vi "3090仪器参数上传.vi"(11 "错误输入（无错误）":errorcluster) -> (15 "error out":errorcluster)   [LabVIEW 2016, in "数据传输系统.lvlib"]
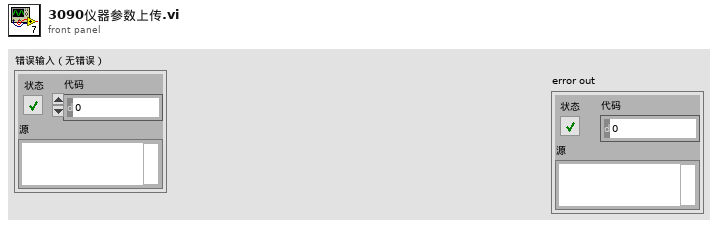
[diagram p1: front panel]
types:
  T1 = cluster{"氨氮仪器参数索引起始时间":string, "总磷仪器参数索引起始时间":string, "总氮仪器参数索引起始时间":string, "CODMn仪器参数索引起始时间":string, "CODCr仪器参数索引起始时间":string, "DO仪器参数索引起始时间":string, "PH仪器参数索引起始时间":string, "比电导率仪器参数索引起始时间":string, "水温仪器参数索引起始时间":string, "浊度仪器参数索引起始时间":string, "叶绿素a仪器参数索引起始时间":string, "藻密度仪器参数索引起始时间":string, "ORP仪器参数索引起始时间":string, "氟化物仪器参数索引起始时间":string, "挥发酚仪器参数索引起始时间":string}
  T2 = cluster{"[0]":string, "[1]":string, "[2]":string, "[3]":string, "[4]":string, "[5]":string, "[6]":string, "[7]":string, "[8]":string, "[9]":string, "[10]":string, "[11]":string, "[12]":string, "[13]":string, "[14]":string}
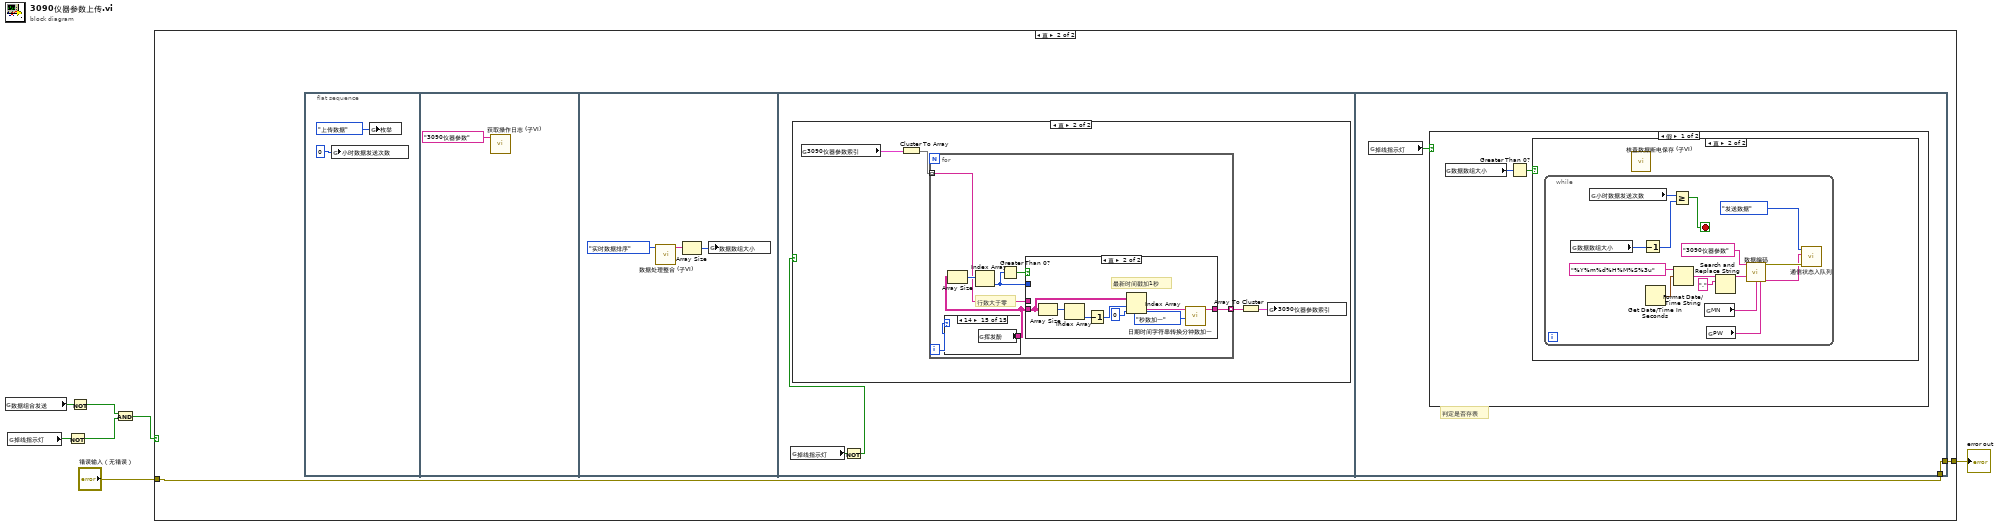
[diagram p0: block diagram]
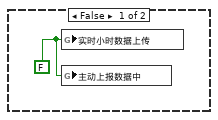
[diagram p2: hidden frame]
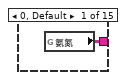
[diagram p4: hidden frame]
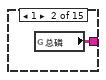
[diagram p5: hidden frame]
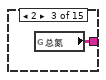
[diagram p6: hidden frame]
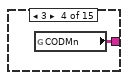
[diagram p7: hidden frame]
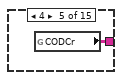
[diagram p8: hidden frame]
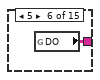
[diagram p9: hidden frame]
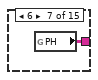
[diagram p10: hidden frame]
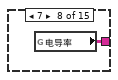
[diagram p11: hidden frame]
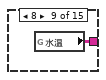
[diagram p12: hidden frame]
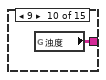
[diagram p13: hidden frame]
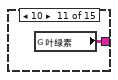
[diagram p14: hidden frame]
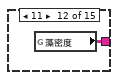
[diagram p15: hidden frame]
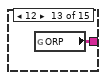
[diagram p16: hidden frame]
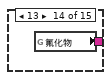
[diagram p17: hidden frame]
diagram:
  n1 = global read "断电保存全局.vi" "数据组合发送"() -> (w4:bool)
  n2 = global read "全局 数据发送重叠.vi" "掉线指示灯"() -> (w7:bool)
  n3 = Not(x=w7) -> (.not. x?=w2:bool)
  n4 = Not(x=w4) -> (.not. x?=w3:bool)
  n5 = And(x=w3, y=w2) -> (x .and. y?=w1:bool)
  n6 = case shown="真" w1 {
    tunnel: [_ w10] -> w6
    tunnel: "错误输入（无错误）" -> [_ w9]
    frame False {
      w8 = FALSE ("小时数据上传")
      n7 = global write "全局1.vi" "实时小时数据上传"(w8) -> ()
      n8 = global write "全局 数据发送重叠.vi" "主动上报数据中"(w8) -> ()
    }
    frame True {
      n9 = flat-sequence {
        tunnel: [w54] -> w10
        tunnel: w9 -> [w54]
        frame #0 {
          n10 = global write "全局 小时数据发送次数.vi" "小时数据发送次数"(0 ("小时数据发送次数")) -> ()
          n11 = global write "全局1.vi" "枚举"(enum16{"返回请求应答", "上传数据", "返回执行结果"}."上传数据" ("枚举")) -> ()
        }
        frame #1 {
          n12 = call "获取操作日志 (子VI).vi"("table输入"="3090仪器参数") -> ()  [unwired: 11 in]
        }
        frame #2 {
          n13 = call "数据处理整合 (子VI).vi"("枚举"=enum16{"实时数据排序", "小时数据排序"}."实时数据排序") -> ("已排序的数组"=w16:string[])  [unwired: 10 in]
          n14 = Array Size(array=w16) -> (size(s)=w15:i32)
          n15 = global write "全局 数据数组大小.vi" "数据数组大小"(w15) -> ()
        }
        frame #3 {
          n16 = global read "全局 数据发送重叠.vi" "掉线指示灯"() -> (w18:bool)
          n17 = Not(x=w18) -> (.not. x?=w17:bool)
          n18 = case shown="真" w17 {
            frame False {
            }
            frame True {
              n19 = global read "全局 时间2.vi" "3090仪器参数索引"() -> (w22:T1)
              n20 = Cluster To Array(cluster=w22) -> (array=w21:string[])
              n21 = for {
                tunnel: [w26] -> w19 mode=indexing
                tunnel: w21 -> [w25] mode=indexing
                i -> [w24]
                # "行数大于零"
                n22 = case shown="14" w24 {
                  tunnel: [w30 w31 w32 w33 w34 w35 w36 w37 w38 w39 w40 w41 w42 w43 w44] -> w23
                  frame 0, Default {
                    n23 = global read "全局 所有参数.vi" "氨氮"() -> (w30:string[][])
                  }
                  frame 1 {
                    n24 = global read "全局 所有参数.vi" "总磷"() -> (w31:string[][])
                  }
                  frame 2 {
                    n25 = global read "全局 所有参数.vi" "总氮"() -> (w32:string[][])
                  }
                  frame 3 {
                    n26 = global read "全局 所有参数.vi" "CODMn"() -> (w33:string[][])
                  }
                  frame 4 {
                    n27 = global read "全局 所有参数.vi" "CODCr"() -> (w34:string[][])
                  }
                  frame 5 {
                    n28 = global read "全局 所有参数.vi" "DO"() -> (w35:string[][])
                  }
                  frame 6 {
                    n29 = global read "全局 所有参数.vi" "PH"() -> (w36:string[][])
                  }
                  frame 7 {
                    n30 = global read "全局 所有参数.vi" "电导率"() -> (w37:string[][])
                  }
                  frame 8 {
                    n31 = global read "全局 所有参数.vi" "水温"() -> (w38:string[][])
                  }
                  frame 9 {
                    n32 = global read "全局 所有参数.vi" "浊度"() -> (w39:string[][])
                  }
                  frame 10 {
                    n33 = global read "全局 所有参数.vi" "叶绿素"() -> (w40:string[][])
                  }
                  frame 11 {
                    n34 = global read "全局 所有参数.vi" "藻密度"() -> (w41:string[][])
                  }
                  frame 12 {
                    n35 = global read "全局 所有参数.vi" "ORP"() -> (w42:string[][])
                  }
                  frame 13 {
                    n36 = global read "全局 所有参数.vi" "氟化物"() -> (w43:string[][])
                  }
                  frame 14 {
                    n37 = global read "全局 所有参数.vi" "挥发酚"() -> (w44:string[][])
                  }
                }
                n38 = Array Size(array=w23) -> (size(s)=w28:i32[])
                n39 = Index Array(array=w28) -> (element=w27:i32)  [unwired: 1 in]
                n40 = Greater Than 0?(x=w27) -> (x > 0?=w29:bool)
                n41 = case shown="真" w29 {
                  tunnel: w27 -> [_ _]
                  tunnel: w23 -> [_ w50]
                  tunnel: [w45 w47] -> w26
                  tunnel: w25 -> [w45 _]
                  frame False {
                  }
                  frame True {
                    # "最新时间戳加1秒"
                    n42 = Array Size(array=w50) -> (size(s)=w52:i32[])
                    n43 = Index Array(array=w52) -> (element=w51:i32)  [unwired: 1 in]
                    n44 = Decrement(x=w51) -> (x-1=w49:i32)
                    n45 = Index Array(array=w50, index (row)=w49, index (col)=0 ("禁用的索引 (列)")) -> (element=w53:string)
                    n46 = call "日期时间字符串转换分钟数加一.vi"("枚举"=enum16{"分钟数加一", "秒数加一", "小时数加一"}."秒数加一", "data[0]"=w53) -> ("日期/时间字符串"=w47:string)  [unwired: 9 in]
                  }
                }
              }
              n47 = Array To Cluster(array=w19) -> (cluster=w20:T2)
              n48 = global write "全局 时间2.vi" "3090仪器参数索引"(w20) -> ()
            }
          }
        }
        frame #4 {
          # "判定是否存表"
          n49 = global read "全局 数据发送重叠.vi" "掉线指示灯"() -> (w55:bool)
          n50 = case shown="假" w55 {
            frame False {
              n51 = global read "全局 数据数组大小.vi" "数据数组大小"() -> (w56:i32)
              n52 = Greater Than 0?(x=w56) -> (x > 0?=w57:bool)
              n53 = case shown="真" w57 {
                frame False {
                }
                frame True {
                  n54 = while {
                    stop <- w60 stop-if-true
                    n55 = global read "全局 数据数组大小.vi" "数据数组大小"() -> (w62:i32)
                    n56 = global read "全局 小时数据发送次数.vi" "小时数据发送次数"() -> (w63:i32)
                    n57 = Decrement(x=w62) -> (x-1=w61:i32)
                    n58 = Get Date/Time In Seconds() -> (seconds since 1Jan1904=w70:timestamp)
                    n59 = Greater Or Equal?(x=w63, y=w61) -> (x >= y?=w60:bool)
                    n60 = Format Date/Time String(time format string (%c)="%Y%m%d%H%M%S%3u" ("时间格式字符串(%c)"), seconds (now)=w70) -> (date/time string=w69:string)  [unwired: 1 in]
                    n61 = global read "断电保存全局.vi" "MN"() -> (w66:string)
                    n62 = global read "断电保存全局.vi" "PW"() -> (w65:string)
                    n63 = Search and Replace String(input string=w69, search string="." ("搜索字符串")) -> (result string=w67:string)  [unwired: 6 in, 3 out]
                    n64 = call "数据编码.vi"("table输入"="3090仪器参数" ("新元素/子数组"), "QN"=w67, "MN"=w66, "PW"=w65) -> ("错误常量"=w64:errorcluster, "通讯包字符串"=w58:string)  [unwired: 10 in]
                    n65 = call "通信状态入队列.vi"("错误输入（无错误）"=w64, "发送报文"=w58, "枚举"=enum16{"打开连接", "发送数据", "读取数据", "数据处理", "关闭连接"}."发送数据") -> ()  [unwired: 8 in, 1 out]
                  }
                  n66 = call "核查数据断电保存 (子VI).vi"() -> ()  [unwired: 12 in]
                }
              }
            }
            frame True {
            }
          }
        }
      }
    }
  }
  "error out" <- w6
